vi "Validate Arguments.vi"(8 "error in (no error)":errorcluster, 11 "GPackCLI in":refnum<class "GPackCLI.lvclass">) -> (0 "error out":errorcluster, 3 "GPackCLI out":refnum<class "GPackCLI.lvclass">)   [LabVIEW 2020, in "GPackTools.lvlib" / "GPackCLI.lvclass"]
uses:
  GPackCLI.lvclass
  GPackCLI.lvclass/GPackCLI.ctl
  CLIAction/CLIAction.lvclass
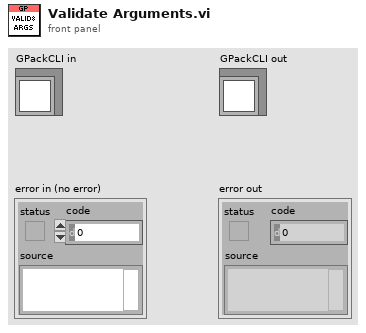
[diagram p1: front panel]
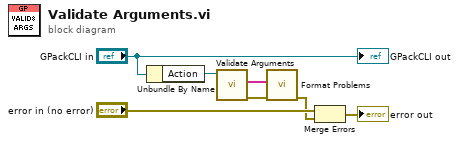
[diagram p0: block diagram]
diagram:
  n1 = Unbundle By Name("GPackCLI in") -> ("Action"=w5:refnum<class "CLIAction.lvclass">)
  n2 = call-dynamic "Validate Arguments.vi"("CLIAction in"=w5) -> ("error out"=w2:errorcluster, "Problems"=w3:string[])  [unwired: 8 in, 1 out]
  n3 = call "Format Problems.vi"("error in (no error)"=w2, "Problems"=w3) -> ("error out"=w1:errorcluster)  [unwired: 9 in]
  n4 = Merge Errors("error in (no error)", w1) -> (→"error out":errorcluster)
  "GPackCLI out" <- "GPackCLI in"
